vi "Import Configuration.vi"(8 "error in":errorcluster, 10 "configuration file path":path, 11 "data sharing framework custom device":T1 format="%.0x") -> (0 "error out":errorcluster, 3 "data sharing framework custom device":T1 format="%.0x")   [LabVIEW 2020, in "Data Sharing Framework Custom Device Scripting.lvlib"]
doc: "Within the system definition, updates an existing instance of the Data Sharing Framework custom device based on the information in the input configuration file (.dsf)."
uses:
  Data Sharing Framework Custom Device Scripting.lvlib
  <vilib>/NI VeriStand/Custom Device API/Custom Device Item Ref.ctl
  System Explorer/DSF System Explorer.lvlib
  Includes/DSF Core.lvlibp/Classes/Configuration Session/Configuration Session.lvclass
  <vilib>/NI VeriStand/Custom Device API/Custom Device API.lvlib
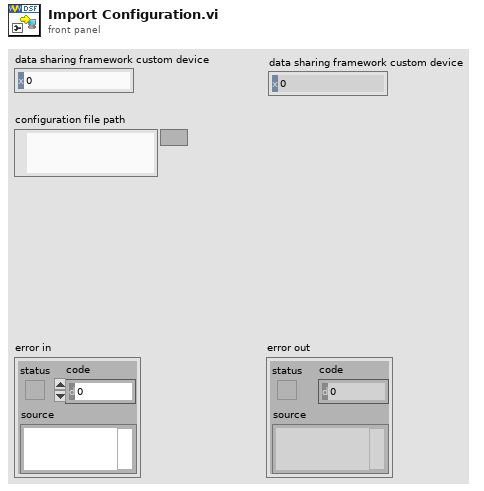
[diagram p1: front panel]
types:
  T1 = typedef "Custom Device API.lvlib/Custom Device Item Ref.ctl" = u64
  T2 = typedef "DSF Core.lvlibp/DSF Version Info.ctl" = cluster{"major":u32, "minor":u32, "fix":u32, "build":string}
  T3 = typedef "DSF Core.lvlibp/DSF Engine Framework Configuration.ctl" = cluster{"plugins":T4[]}
  T4 = typedef "DSF Core.lvlibp/DSF Engine Plugin Configuration.ctl" = cluster{"core":T5, "component settings":T7[], "threads":T8[]}
  T5 = typedef "DSF Core.lvlibp/Plugin Configuration.lvclass/Core Plugin Configuration.ctl" = cluster{"name":string, "components":string[], "cycle timing":T6}
  T6 = typedef "DSF Core.lvlibp/DSF Timing Info.ctl" = cluster{"priority":u64, "decimation":u64, "offset":u64}
  T7 = typedef "DSF Core.lvlibp/DSF Settings Info.ctl" = cluster{"component":string, "values":cluster{"key":string, "value":string}[]}
  T8 = typedef "DSF Core.lvlibp/DSF Engine Plugin Thread Configuration.ctl" = cluster{"core":T9, "component settings":T7[], "transfer groups":T10[]}
  T9 = typedef "DSF Core.lvlibp/Thread Configuration.lvclass/Core Thread Configuration.ctl" = cluster{"processor":i32, "priority offset":i16}
  T10 = typedef "DSF Core.lvlibp/DSF Engine Transfer Group Configuration.ctl" = cluster{"core":T11, "component settings":T7[], "transfers":T14[]}
  T11 = typedef "DSF Core.lvlibp/Group Configuration.lvclass/Core Group Configuration.ctl" = cluster{"name":string, "direction":T12, "cycle timing":T6, "timeout behavior":T13, "enable conversion":bool}
  T12 = typedef "DSF Core.lvlibp/DSF Direction.ctl" = enum8{"Tx", "Rx"}
  T13 = typedef "DSF Core.lvlibp/DSF Timeout Behavior.ctl" = enum8{"Increment Late Count", "Throw Error"}
  T14 = typedef "DSF Core.lvlibp/DSF Engine Transfer Configuration.ctl" = cluster{"core":T15, "component settings":T7[], "channels":T16[]}
  T15 = typedef "DSF Core.lvlibp/Transfer Configuration.lvclass/Core Transfer Configuration.ctl" = cluster{"name":string}
  T16 = typedef "DSF Core.lvlibp/DSF Engine Channel Configuration.ctl" = cluster{"core":T17, "component settings":T7[]}
  T17 = typedef "DSF Core.lvlibp/Channel Configuration.lvclass/Core Channel Configuration.ctl" = cluster{"name":string, "units":string, "engine data type":T18, "string data type":T18, "string offset":u64}
  T18 = typedef "DSF Core.lvlibp/DSF Data Type.ctl" = enum8{"Bool", "SGL", "DBL", "I8", "I16", "I32", "I64", "U8", "U16", "U32", "U64"}
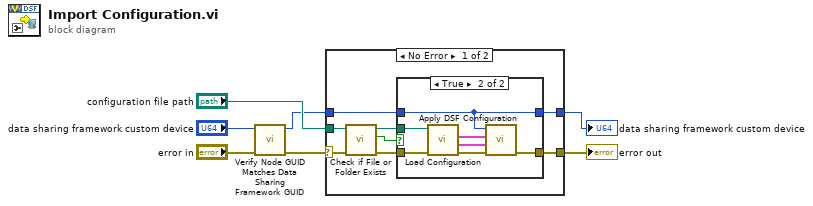
[diagram p0: block diagram]
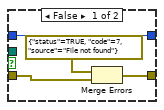
[diagram p2: hidden frame]
diagram:
  n1 = call "Verify Node GUID Matches Data Sharing Framework GUID.vi"("error in"="error in", "data sharing framework custom device in"="data sharing framework custom device") -> ("error out"=w3:errorcluster, "data sharing framework custom device out"=w1:T1)  [unwired: 8 in]
  n2 = case shown="No Error" w3 {
    selector: w3 -> [w11 w28]
    tunnel: [w14 w28] -> w7
    tunnel: w1 -> [w15 w27]
    tunnel: "configuration file path" -> [w12 _]
    tunnel: [w13 w27] -> w5
    frame No Error {
      n3 = call <vilib>:"Check if File or Folder Exists.vi"("error in (no error)"=w11, "path"=w12) -> ("error out"=w10:errorcluster, "file or folder exists?"=w8:bool, "dup path"=w9:path)  [unwired: 7 in]
      n4 = case shown="True" w8 {
        tunnel: w9 -> [_ w26]
        tunnel: w15 -> [w19 w20]
        tunnel: w10 -> [w18 w23]
        tunnel: [w17 w21] -> w14
        tunnel: [w19 w20] -> w13
        frame False {
          n5 = Merge Errors(errorcluster {"status"=TRUE, "code"=7, "source"="File not found"}, w18) -> (w17:errorcluster)
        }
        frame True {
          n6 = call "Load Configuration.vi"("error in (no error)"=w23, "configuration file path"=w26) -> ("error out"=w22:errorcluster, "version"=w24:T2, "framework configuration"=w25:T3)  [unwired: 6 in, 1 out]
          n7 = call "Apply DSF Configuration.vi"("error in (no error)"=w22, "version"=w24, "framework configuration"=w25, "Item Ref in"=w20) -> ("error out"=w21:errorcluster)  [unwired: 7 in]
        }
      }
    }
    frame Error {
    }
  }
  "data sharing framework custom device" <- w5
  "error out" <- w7
